vi "Test Process Generate Broadcast Event.vi"(8 "error in (no error)":errorcluster, 11 "Process Test In":refnum<class "Process Test.lvclass">) -> (0 "error out":errorcluster, 3 "Process Test Out":refnum<class "Process Test.lvclass">)   [LabVIEW 2020, in "Process Test.lvclass"]
uses:
  Process Test.lvclass
  C:/Program Files (x86)/National Instruments/LabVIEW 2020/vi.lib/Asteme/LUnit/Test Case.lvclass
  Mock Process/Mock Process.lvclass
  C:/Users/anton/Documents/GitHub/Triarc-Framework/source/Framework/Process/Process.lvclass
  Framework/Process/Process.lvclass/Process.ctl
  <vilib>/Asteme/LUnit/Test Case.lvclass/Test Case.ctl
  <vilib>/Asteme/LUnit/LUnit Assertion Result.lvclass/LUnit Assertion Result.ctl
  Framework/Process/Public/Get Lifecycle State.vi
  Framework/Process/Private/SubVIs/Wait for finish.vi
  Framework/Process/Protected/Messaging/Enqueue Message.vi
  Framework/Process/Private/SubVIs/Set Lifecycle State.vi
  <vilib>/Asteme/LUnit/Palette/Pass If.vi
  <vilib>/Asteme/LUnit/Set Assertion Type.vi
  <vilib>/Asteme/LUnit/Palette/Pass.vi
  <vilib>/Asteme/LUnit/Palette/Fail.vi
  <vilib>/Asteme/LUnit/Variant to string.vi
  <vilib>/Utility/error.llb/Clear Errors.vi
  <vilib>/Asteme/LUnit/LUnit Write Assertion Type.vi
  <vilib>/Asteme/LUnit/Add test result.vi
  <vilib>/Asteme/LUnit/LUnit Write Passed.vi
  <vilib>/Asteme/LUnit/LUnit Get Test Case.vi
  <vilib>/Asteme/LUnit/LUnit Write Message.vi
  <vilib>/Asteme/LUnit/LUnit Write Description.vi
  <vilib>/Asteme/LUnit/Read Test Case Name.vi
  <vilib>/Utility/error.llb/Error Cluster From Error Code.vi
  <vilib>/Asteme/LUnit/Assertion Result/LUnit Get Test Name.vi
  <vilib>/Utility/Data Type/Get Type Information.vi
  <vilib>/Utility/LVClass/Get LV Class Name.vi
  <vilib>/Asteme/LUnit/LUnit Assertion Result.lvclass
  Framework/Process/Process.lvclass
  <vilib>/Asteme/LUnit/Test Case.lvclass
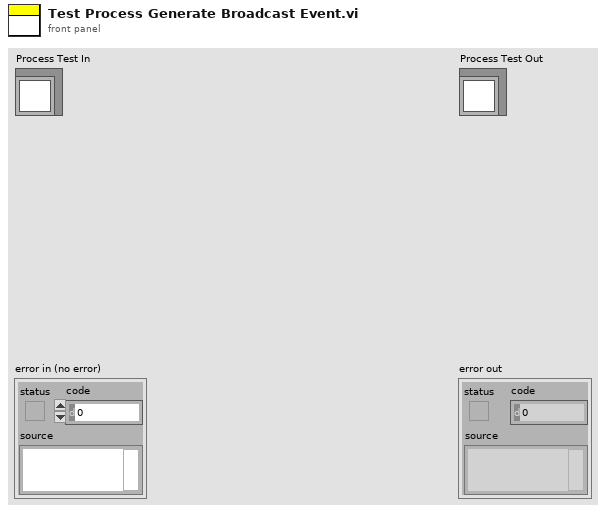
[diagram p1: front panel]
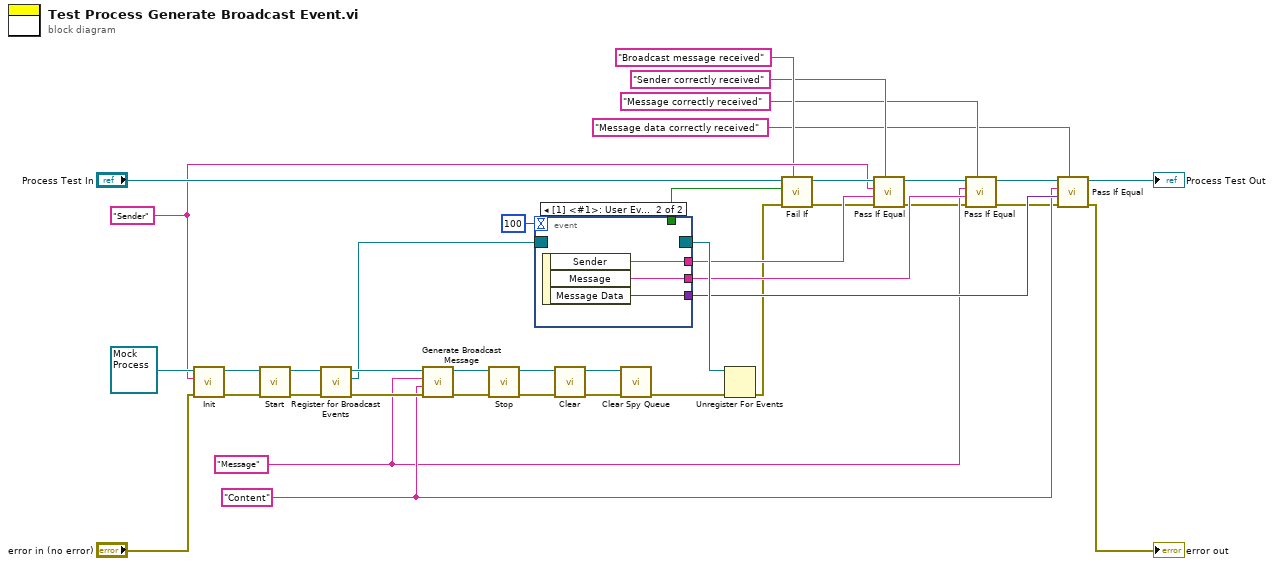
[diagram p0: block diagram]
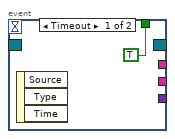
[diagram p2: hidden frame]
diagram:
  w13 = "Sender" ("Message")
  w15 = "Content" ("Message")
  w14 = "Message" ("Message")
  n1 = call-dynamic "Init.vi"("error in (no error)"="error in (no error)", "Name"=w13, "Mock Process In"=refnum<class "Mock Process.lvclass"> refnum ("Mock Process.lvclass")) -> ("error out"=w37:errorcluster, "Mock Process Out"=w38:refnum<class "Mock Process.lvclass">)  [unwired: 7 in]
  n2 = call "Start.vi"("error in (no error)"=w37, "Process In"=w38) -> ("error out"=w26:errorcluster, "Process Out"=w28:refnum<class "Mock Process.lvclass">)  [unwired: 8 in]
  n3 = call-dynamic "Register for Broadcast Events.vi"("error in (no error)"=w26, "Process In"=w28) -> ("error out"=w25:errorcluster, "Event Registration Refnum"=w24:refnum<event-registration>, "Process Out"=w27:refnum<class "Mock Process.lvclass">)  [unwired: 7 in]
  n4 = call "Generate Broadcast Message.vi"("error in (no error)"=w25, "Message Data"=w15, "Message"=w14, "Mock Process In"=w27) -> ("error out"=w35:errorcluster, "Mock Process Out"=w36:refnum<class "Mock Process.lvclass">)  [unwired: 6 in]
  n5 = call "Stop.vi"("error in (no error)"=w35, "Process In"=w36) -> ("error out"=w33:errorcluster, "Process Out"=w34:refnum<class "Mock Process.lvclass">)  [unwired: 7 in, 1 out]
  n6 = event shown="[1] <#1>: User Event" {
    selector: w24 -> [_ _]
    dyn-events: [_ _] -> w23
    timeout: 100 -> [_ _]
    tunnel: [TRUE _] -> w20
    tunnel: [_ w43] -> w18
    tunnel: [_ w42] -> w17
    tunnel: [_ w41] -> w16
    event Timeout {
      n7 = event-data() -> ()  [unwired: 1 in, 3 out]
    }
    event User Event {
      n8 = event-data() -> ("Sender"=w43:string, "Message"=w42:string, "Message Data"=w41:variant)  [unwired: 1 in]
    }
  }
  n9 = call-dynamic "Clear.vi"("error in (no error)"=w33, "Mock Process In"=w34) -> ("error out"=w31:errorcluster, "Mock Process Out"=w32:refnum<class "Mock Process.lvclass">)  [unwired: 8 in]
  n10 = call-dynamic "Clear Spy Queue.vi"("error in (no error)"=w31, "Mock Process In"=w32) -> ("error out"=w22:errorcluster)  [unwired: 8 in, 1 out]
  n11 = Unregister For Events(event registration refnum=w23, error in=w22) -> (error out=w7:errorcluster)
  n12 = call <vilib>:"Fail If.vi"("Description"="Broadcast message received", "error in (no error)"=w7, "Fail?"=w20, "Test Case In"="Process Test In") -> ("error out"=w12:errorcluster, "Test Case Out"=w21:refnum<class "Process Test.lvclass">)  [unwired: 6 in]
  n13 = call <vilib>:"Pass If Equal.vi"("Description"="Sender correctly received", "error in (no error)"=w12, "Actual"=w18, "Expected"=w13, "Test Case In"=w21) -> ("error out"=w10:errorcluster, "Test Case Out"=w11:refnum<class "Process Test.lvclass">)  [unwired: 5 in]
  n14 = call <vilib>:"Pass If Equal.vi"("Description"="Message correctly received", "error in (no error)"=w10, "Actual"=w17, "Expected"=w14, "Test Case In"=w11) -> ("error out"=w8:errorcluster, "Test Case Out"=w9:refnum<class "Process Test.lvclass">)  [unwired: 5 in]
  n15 = call <vilib>:"Pass If Equal.vi"("Description"="Message data correctly received", "error in (no error)"=w8, "Actual"=w16, "Expected"=w15, "Test Case In"=w9) -> ("error out"=→"error out":errorcluster, "Test Case Out"=→"Process Test Out":refnum<class "Process Test.lvclass">)  [unwired: 5 in]
